vi "Read Binary Config.vi"(4 "Class Name is Included":bool, 6 "byte order (0:big-endian, network order)":T1(ring), 8 "error in (no error)":errorcluster, 10 "Binary":string, 11 "Concatenate_STR in":refnum<class "Concatenate_STR.lvclass">) -> (0 "error out":errorcluster, 2 "Remaining":string, 3 "Concatenate_STR out":refnum<class "Concatenate_STR.lvclass">)   [LabVIEW 2021, in "Concatenate_STR.lvclass"]
uses:
  Concatenate_STR.lvclass
  Concatenate_STR.lvclass/Concatenate_STR.ctl
  Abs_Types/Value/Abs_Value.lvclass
  C:/Program Files (x86)/National Instruments/LabVIEW 2021/vi.lib/TSA/Abstract Data Classes/Abs_Types/Type/Abs_Type.lvclass
  Abs_Types/String/Abs_String.lvclass
  Abs_Types/Type/Abs_Type.lvclass
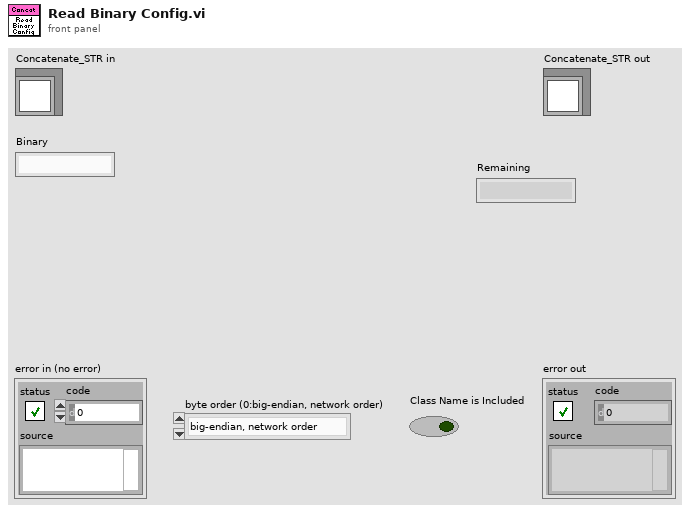
[diagram p1: front panel]
types:
  T1 = enum16{"big-endian, network order", "native, host order", "little-endian"}
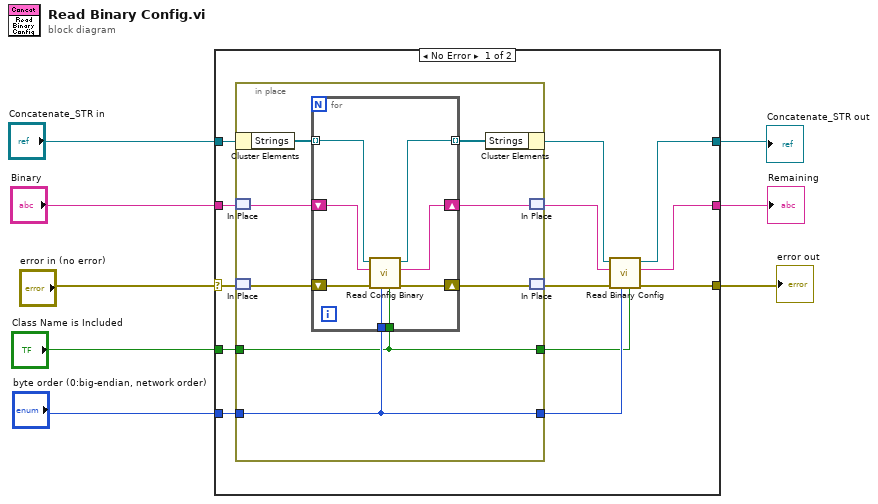
[diagram p0: block diagram]
diagram:
  n1 = case shown="No Error" "error in (no error)" {
    selector: "error in (no error)" -> [w20 w38]
    tunnel: "Binary" -> [w21 w39]
    tunnel: "Concatenate_STR in" -> [w19 w40]
    tunnel: [w15 w38] -> w4
    tunnel: [w14 w40] -> w6
    tunnel: "Class Name is Included" -> [w13 _]
    tunnel: "byte order (0:big-endian, network order)" -> [w12 _]
    tunnel: [w9 w39] -> w5
    frame No Error {
      n2 = in-place {
        in-place-border: w13 -> [w24]
        in-place-border: w12 -> [w25]
        in-place-border: [w25] -> w11
        in-place-border: [w24] -> w10
        n3 = in-place-cluster #1(w19) -> ("Strings"=w28:refnum<class "Abs_Value.lvclass">[])
        n4 = in-place-match #2(w21) -> (w23:string)
        n5 = in-place-match #3(w20) -> (w29:errorcluster)
        n6 = for {
          tunnel: w28 -> [w36] mode=indexing
          tunnel: [w35] -> w27 mode=indexing
          tunnel: w25 -> [w33]
          tunnel: w24 -> [w32]
          shift-right: [w34] -> w26
          shift-left: w29 -> [w37]
          shift-right: [w30] -> w22
          shift-left: w23 -> [w31]
          n7 = call "Read Config Binary.vi"("Class Name is Included"=w32, "byte order (0:big-endian, network order)"=w33, "error in (no error)"=w37, "Binary"=w31, "Abs_Type in"=w36) -> ("error out"=w34:errorcluster, "Remaining"=w30:string, "Abs_Type out"=w35:refnum<class "Abs_Value.lvclass">)  [unwired: 4 in]
        }
        n8 = in-place-cluster #1("Strings"=w27) -> (w16:refnum<class "Concatenate_STR.lvclass">)
        n9 = in-place-match #2(w22) -> (w17:string)
        n10 = in-place-match #3(w26) -> (w18:errorcluster)
      }
      n11 = call-parent "Read Binary Config.vi"("Class Name is Included"=w10, "byte order (0:big-endian, network order)"=w11, "error in (no error)"=w18, "Binary"=w17, "Abs_Type in"=w16) -> ("error out"=w15:errorcluster, "Remaining"=w9:string, "Abs_Type out"=w14:refnum<class "Concatenate_STR.lvclass">)  [unwired: 4 in]
    }
    frame Error {
    }
  }
  "error out" <- w4
  "Concatenate_STR out" <- w6
  "Remaining" <- w5
